vi "U3 Stream Example LJ_swSLEEP.vi"() -> ()   [LabVIEW 2021]
panel:
  in  "Resolution Index":u8
  out "Waveform Graph":dbl[][](graph)
  out "# Skipped Scans":i32
  in  "Simulated Processing Delay [ms]":u32
  out "UD Backlog [%]":dbl format="%.2f"
  in  "Scan List":u8[](array[numeric])=[0, 1, 2, 3]
  out "Actual Scan Rate (Hz)":dbl=1000.0 format="%.3f"
  out "ms Per Loop":u32
  out "U3 Backlog [%]":dbl format="%.2f"
  out "Scans Retrieved Sec (measured)":dbl format="%.2f"
  out "# Scans Read":i32
  out "# of iterations":i32
  out "Data":dbl[][](array[numeric]) format="%.3f"
  in  "Scan Rate (Hz)":dbl=1000.0 format="%.3f"
  in  "Data File Extension":string="dat"
  out "Current Data File":path
  in  "Data File Prefix":string="data"
  in  "Write To File":bool
  in  "FirstFound":bool=TRUE
  in  "stop":bool
  in  "Address":string="1"
  out "Error Message":string
  # "Streams using the SLEEP wait mode.  Streaming\nrequires U3 hardware revision 1.21."
  # "The actual scans/sec is controlled\nby hardware and is known.  This\n\"measured\" suggests the rate at\nwhich data is being retreived."
  # "0=Auto"
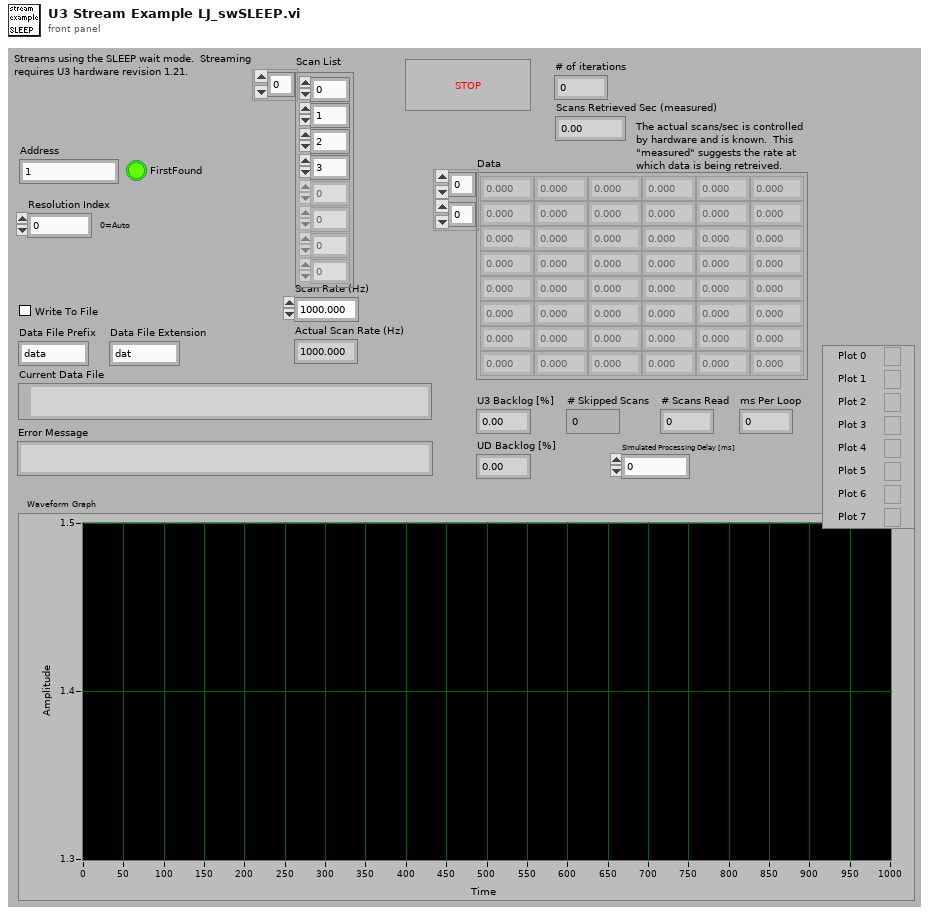
[diagram p1: front panel]
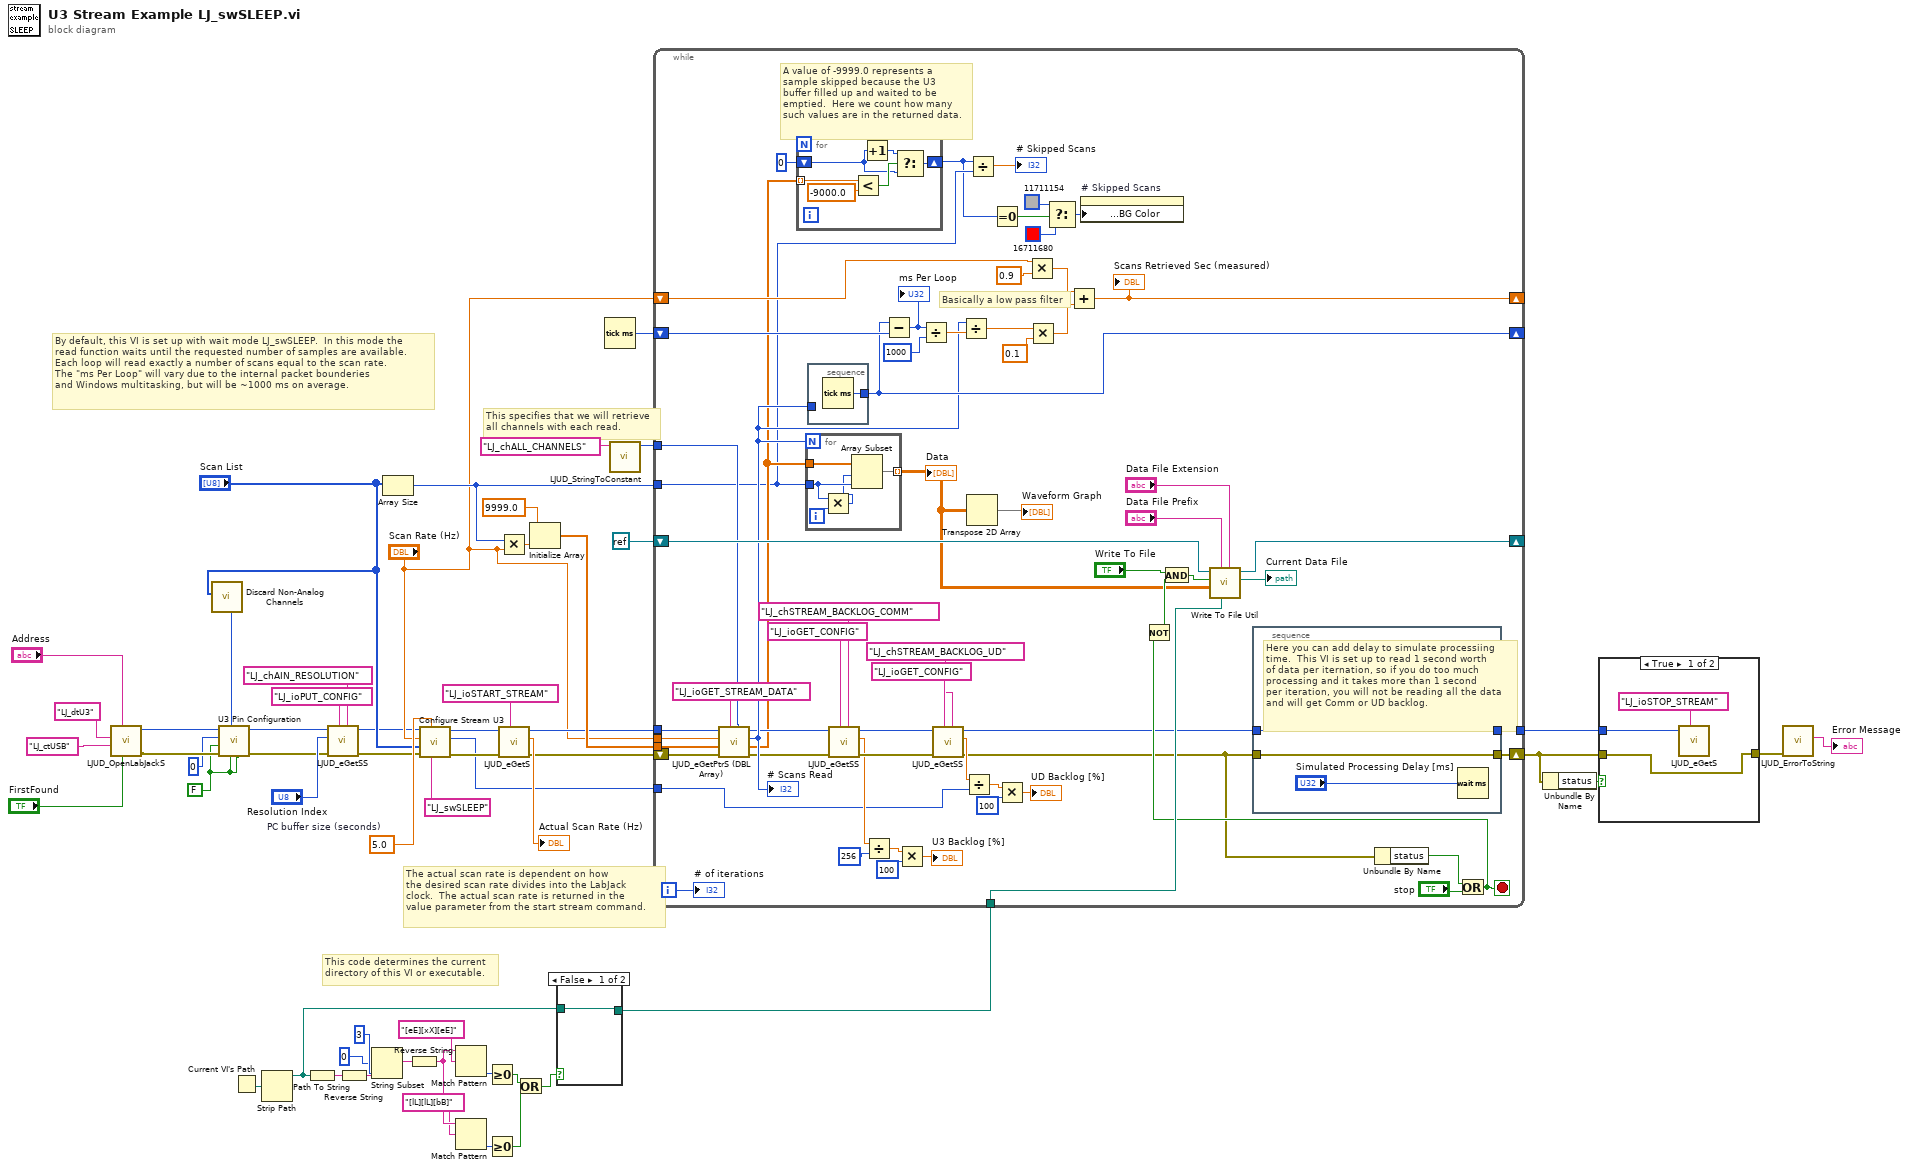
[diagram p0: block diagram]
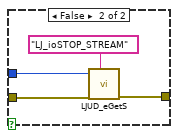
[diagram p2: hidden frame]
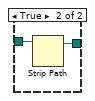
[diagram p3: hidden frame]
diagram:
  w11 = FALSE ("Enable DAC1")
  w25 = 5.0  # PC buffer size (seconds)
  # "This specifies that we will retrieve\nall channels with each read."
  # "The actual scan rate is dependent on how\nthe desired scan rate divides into the LabJack\nclock.  The actual scan rate is returned in the\nvalue parameter from the start stream command."
  # "By default, this VI is set up with wait mode LJ_swSLEEP.  In this mode the\nread function waits until the requested number of samples are available.\nEach loop will read exactly a number of scans equal to the scan rate.\nThe \"ms Per Loop\" will vary due to the internal packet bounderies\nand Windows multitasking, but will be ~1000 ms on average."
  # "This code determines the current\ndirectory of this VI or executable."
  n1 = call "LJUD_OpenLabJackS.vi"("FirstFound"="FirstFound", "Address"="Address", "ConnectionType"="LJ_ctUSB", "DeviceType"="LJ_dtU3") -> ("error out"=w14:errorcluster, "Handle"=w15:i32)  [unwired: 5 in, 1 out]
  n2 = call "Discard Non-Analog Channels.vi"("Channels In"="Scan List") -> ("FIO/EIO Analog Enable"=w10:i32)  [unwired: 7 in, 3 out]
  n3 = call "U3 Pin Configuration.vi"("Enable Counter1"=w11, "Enable Counter0"=w11, "FIO/EIO Analog Enable"=w10, "error in"=w14, "Enable DAC1"=w11, "Number of Timers Enabled"=u8 0, "Handle In"=w15) -> ("error out"=w4:errorcluster, "Handle Out"=w5:i32)  [unwired: 3 in]
  n4 = Current VI's Path() -> (path=w53:path)
  n5 = Strip Path(path=w53) -> (stripped path=w45:path)  [unwired: 1 out]
  n6 = Path To String(path=w45) -> (string=w52:string)
  n7 = call "LJUD_eGetSS.vi"("Channel"="LJ_chAIN_RESOLUTION", "IOType"="LJ_ioPUT_CONFIG", "error in"=w4, "Value Write"="Resolution Index", "Handle In"=w5) -> ("error out"=w3:errorcluster, "Handle Out"=w2:i32)  [unwired: 4 in, 1 out]
  n8 = Reverse String(1:w52) -> (0:w51:string)
  n9 = String Subset(string=w51, offset (0)=0, length (rest)=3 ("length")) -> (substring=w48:string)
  n10 = Array Size(array="Scan List") -> (size(s)=w31:i32)
  n11 = Reverse String(1:w48) -> (0:w44:string)
  n12 = call "Configure Stream U3.vi"("Wait Mode"="LJ_swSLEEP" ("Wait Mode (2)"), "PC buffer size (seconds)"=w25, "error in"=w3, "Scan List (+)"="Scan List", "Scan Rate (Hz)"="Scan Rate (Hz)", "Handle In"=w2) -> ("error out"=w35:errorcluster, "PC buffer size (samples)"=w16:i32, "Handle Out"=w36:i32)  [unwired: 3 in]
  n13 = Match Pattern(string=w44, regular expression="[eE][xX][eE]") -> (offset past match=w46:i32)  [unwired: 1 in, 3 out]
  n14 = Match Pattern(string=w44, regular expression="[lL][lL][bB]") -> (offset past match=w41:i32)  [unwired: 1 in, 3 out]
  n15 = Greater Or Equal To 0?(x=w46) -> (x >= 0?=w42:bool)
  n16 = Greater Or Equal To 0?(x=w41) -> (x >= 0?=w40:bool)
  n17 = Multiply(x=w31, y="Scan Rate (Hz)") -> (x*y=w34:dbl)
  n18 = call "LJUD_eGetS.vi"("IOType"="LJ_ioSTART_STREAM", "error in"=w35, "Handle In"=w36) -> ("error out"=w18:errorcluster, "Value Read"=→"Actual Scan Rate (Hz)":dbl, "Handle Out"=w23:i32)  [unwired: 6 in]
  n19 = Or(x=w42, y=w40) -> (x .or. y?=w39:bool)
  n20 = Initialize Array(9999.0, w34) -> (w32:dbl[])
  n21 = case shown="False" w39 {
    tunnel: w45 -> [w57 w59]
    tunnel: [w57 w58] -> w38
    frame False {
    }
    frame True {
      n22 = Strip Path(path=w59) -> (stripped path=w58:path)  [unwired: 1 out]
    }
  }
  n23 = Tick Count (ms)() -> (millisecond timer value=w26:u32)
  n24 = call "LJUD_StringToConstant.vi"("String"="LJ_chALL_CHANNELS") -> ("Constant Number"=w19:i32)  [unwired: 9 in, 1 out]
  n25 = while {
    tunnel: w16 -> [w77]
    shift-left: w18 -> [w85]
    shift-right: [w73] -> w17
    tunnel: w19 -> [w90]
    shift-left: "Scan Rate (Hz)" -> [w98]
    shift-right: [w95] -> _
    shift-left: w26 -> [w107]
    shift-right: [w104] -> _
    tunnel: [w71] -> w29
    tunnel: w31 -> [w68]
    tunnel: w32 -> [w110]
    tunnel: "Scan Rate (Hz)" -> [w109]
    tunnel: w38 -> [w114]
    shift-left: refnum<k0> refnum -> [w120]
    shift-right: [w119] -> _
    tunnel: w23 -> [w112]
    i -> [w108]
    stop <- w113 stop-if-true
    # "A value of -9999.0 represents a\nsample skipped because the U3\nbuffer filled up and waited to be\nemptied.  Here we count how many\nsuch values are in the returned data."
    # "Basically a low pass filter"
    n26 = call "LJUD_eGetPtrS (DBL Array).vi"("Channel"=w90, "IOType"="LJ_ioGET_STREAM_DATA", "error in"=w85, "DBL Array Write"=w110, "Value"=w109, "Handle In"=w112) -> ("error out"=w93:errorcluster, "DBL Array Read"=w70:dbl[], "Value"=w102:i32, "Handle Out"=w94:i32)  [unwired: 2 in]
    "# Scans Read" <- w102
    n27 = for {
      shift-right: [w125] -> w64
      shift-left: 0 -> [w126]
      tunnel: w70 -> [w129] mode=indexing
      n28 = Less?(x=w129, y=-9000.0) -> (x < y?=w127:bool)
      n29 = Increment(x=w126) -> (x+1=w130:i32)
      n30 = Select(t=w130, s=w127, f=w126) -> (s? t:f=w125:i32)
    }
    n31 = for {
      N: w102 -> [_]
      tunnel: w70 -> [w139]
      tunnel: w68 -> [w138]
      tunnel: [w135] -> w60 mode=indexing
      i -> [w137]
      n32 = Multiply(x=w138, y=w137) -> (x*y=w136:i32)
      n33 = Array Subset(array=w139, index=w136, length=w138) -> (w135:dbl[])
    }
    "Data" <- w60
    n34 = stacked-sequence {
      tunnel: w102 -> [_]
      tunnel: [w134] -> w104
      frame #0 {
        n35 = Tick Count (ms)() -> (millisecond timer value=w134:u32)
      }
    }
    n36 = call "LJUD_eGetSS.vi"("Channel"="LJ_chSTREAM_BACKLOG_COMM", "IOType"="LJ_ioGET_CONFIG", "error in"=w93, "Handle In"=w94) -> ("error out"=w86:errorcluster, "Value Read"=w81:dbl, "Handle Out"=w87:i32)  [unwired: 5 in]
    n37 = Divide(x=w81, y=256) -> (x/y=w84:dbl)
    n38 = Subtract(x=w104, y=w107) -> (x-y=w106:u32)
    "ms Per Loop" <- w106
    n39 = Multiply(x=w84, y=100) -> (x*y=→"U3 Backlog [%]":dbl)
    n40 = Divide(x=w106, y=u32 1000) -> (x/y=w103:dbl)
    n41 = call "LJUD_eGetSS.vi"("Channel"="LJ_chSTREAM_BACKLOG_UD", "IOType"="LJ_ioGET_CONFIG", "error in"=w86, "Handle In"=w87) -> ("error out"=w74:errorcluster, "Value Read"=w76:dbl, "Handle Out"=w72:i32)  [unwired: 5 in]
    n42 = Divide(x=w102, y=w103) -> (x/y=w101:dbl)
    n43 = Divide(x=w76, y=w77) -> (x/y=w78:dbl)
    n44 = Transpose 2D Array(2D array=w60) -> (transposed array=→"Waveform Graph":dbl[][])
    n45 = Divide(x=w64, y=w68) -> (x/y=→"# Skipped Scans":dbl)
    n46 = Equal To 0?(x=w64) -> (x = 0?=w63:bool)
    n47 = Multiply(x=w78, y=100) -> (x*y=→"UD Backlog [%]":dbl)
    n48 = Multiply(x=w98, y=0.9) -> (x*y=w97:dbl)
    n49 = Multiply(x=w101, y=0.1) -> (x*y=w96:dbl)
    n50 = Select(t=u32 11711154, s=w63, f=u32 16711680) -> (s? t:f=w62:u32)
    n51 = Add(x=w97, y=w96) -> (x+y=w95:dbl)
    "Scans Retrieved Sec (measured)" <- w95
    n52 = property on="# Skipped Scans" class="DigNum (strict)"("Numeric Text.Text Colors:BG Color"=w62) -> ()  [unwired: 2 in, 2 out]
    n53 = stacked-sequence {
      tunnel: w74 -> [w133]
      tunnel: [w133] -> w73
      tunnel: w72 -> [w132]
      tunnel: [w132] -> w71
      frame #0 {
        # "Here you can add delay to simulate processiing\ntime.  This VI is set up to read 1 second worth\nof data per iternation, so if you do too much\nprocessing and it takes more than 1 second\nper iteration, you will not be reading all the data\nand will get Comm or UD backlog."
        n54 = Wait (ms)(milliseconds to wait="Simulated Processing Delay [ms]") -> ()  [unwired: 1 out]
      }
    }
    n55 = Unbundle By Name(w74) -> ("status"=w123:bool)
    n56 = Or(x=w123, y="stop") -> (x .or. y?=w113:bool)
    n57 = Not(x=w113) -> (.not. x?=w115:bool)
    n58 = And(x="Write To File", y=w115) -> (x .and. y?=w116:bool)
    n59 = call "Write To File Util.vi"("Data File Extension"="Data File Extension", "Working Directory"=w114, "Data File Prefix"="Data File Prefix", "Data"=w60, "Write To File"=w116, "File Refnum In"=w120) -> ("Current Data File"=→"Current Data File":path, "File Refnum Out"=w119:refnum<file>)  [unwired: 3 in, 1 out]
    "# of iterations" <- w108
  }
  n60 = Unbundle By Name(w17) -> ("status"=w21:bool)
  n61 = case shown="True" w21 {
    tunnel: w29 -> [w141 w145]
    tunnel: [w140 w144] -> w28
    tunnel: w17 -> [w140 w143]
    frame True {
      n62 = call "LJUD_eGetS.vi"("IOType"="LJ_ioSTOP_STREAM", "Handle In"=w141) -> ()  [unwired: 7 in, 3 out]
    }
    frame False {
      n63 = call "LJUD_eGetS.vi"("IOType"="LJ_ioSTOP_STREAM", "error in"=w143, "Handle In"=w145) -> ("error out"=w144:errorcluster)  [unwired: 6 in, 2 out]
    }
  }
  n64 = call "LJUD_ErrorToString.vi"("error in"=w28) -> ("String"=→"Error Message":string)  [unwired: 10 in]
